vi "HH_Set.vi"(0 "Device List":T3(array[cluster]), 5 "CFD Settings":T2={"Sync Level"=150, "Sync ZeroX"=10, "Sync Offset"=-8000, "Chan Settings"=[{"CHx Level"=50, "CHx ZeroX"=10, "CHx Offset"=350}, {"CHx Level"=50, "CHx ZeroX"=10, "CHx Offset"=50}, {"CHx Level"=150, "CHx ZeroX"=10, "CHx Offset"=19250}, {"CHx Level"=150, "CHx ZeroX"=10, "CHx Offset"=19500}]}, 11 "error in (no error)":errorcluster, 12 "SyncDiv":i32=8, 13 "Offset":i32) -> (3 "ht3 header out":T1={"Comment"="", "Binning"=0, "Offset"=0, "AcquisitionTime (ms)"=0, "HardwareSerial"=0, "SyncDivider"=0, "Resolution (ps)"=0.0, "InpRate0"=0, "InpRate1"=0, "CFD Settings"={"Sync Level"=150, "Sync ZeroX"=10, "Sync Offset"=-1000, "Chan Settings"=[{"CHx Level"=50, "CHx ZeroX"=10, "CHx Offset"=0}, {"CHx Level"=50, "CHx ZeroX"=10, "CHx Offset"=0}, {"CHx Level"=50, "CHx ZeroX"=10, "CHx Offset"=0}, {"CHx Level"=50, "CHx ZeroX"=10, "CHx Offset"=0}]}, "ModuleInfo"=[], "BaseResolution (ps)"=0.0, "RefClockSource"=0, "ChanInfo"=[], "SyncRate"=0, "InputsEnabled"=0}, 6 "Resolution (ps)":dbl, 8 "Range":i32, 10 "Sync Rate":i32, 15 "error out":errorcluster)   [LabVIEW 2010]
uses:
  hhlib.dll
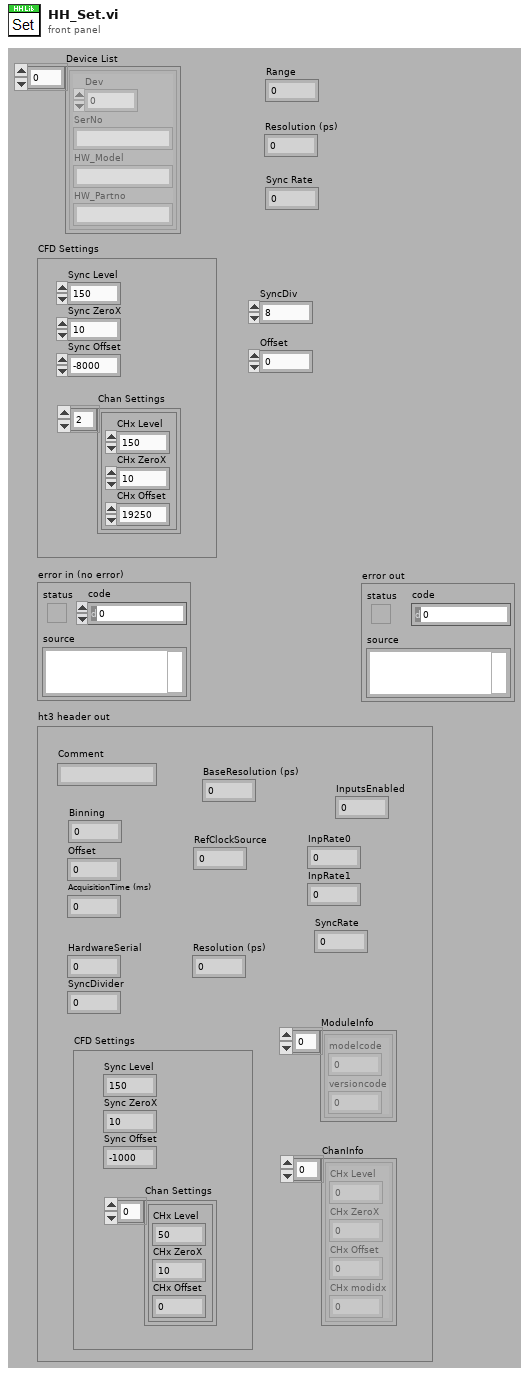
[diagram p1: front panel]
types:
  T1 = cluster{"Comment":string, "Binning":i32, "Offset":i32, "AcquisitionTime (ms)":i32, "HardwareSerial":i32, "SyncDivider":i32, "Resolution (ps)":dbl, "InpRate0":i32, "InpRate1":i32, "CFD Settings":cluster{"Sync Level":i32, "Sync ZeroX":i32, "Sync Offset":i32, "Chan Settings":cluster{"CHx Level":i32, "CHx ZeroX":i32, "CHx Offset":i32}[]}, "ModuleInfo":cluster{"modelcode":i32, "versioncode":i32}[], "BaseResolution (ps)":dbl, "RefClockSource":i32, "ChanInfo":cluster{"CHx Level":i32, "CHx ZeroX":i32, "CHx Offset":i32, "CHx modidx":i32}[], "SyncRate":i32, "InputsEnabled":i64}
  T2 = cluster{"Sync Level":i32, "Sync ZeroX":i32, "Sync Offset":i32, "Chan Settings":cluster{"CHx Level":i32, "CHx ZeroX":i32, "CHx Offset":i32}[]}
  T3 = cluster{"Dev":i32, "SerNo":string, "HW_Model":string, "HW_Partno":string}[]
  T4 = cluster{"CHx Level":i32, "CHx ZeroX":i32, "CHx Offset":i32, "CHx modidx":i32}
  T5 = cluster{"CHx Level":i32, "CHx ZeroX":i32, "CHx Offset":i32}
  T6 = cluster{"CHx Level":i32, "CHx ZeroX":i32, "CHx Offset":i32, "CHx modidx":i32}[]
  T7 = cluster{"CHx Level":i32, "CHx ZeroX":i32, "CHx Offset":i32}[]
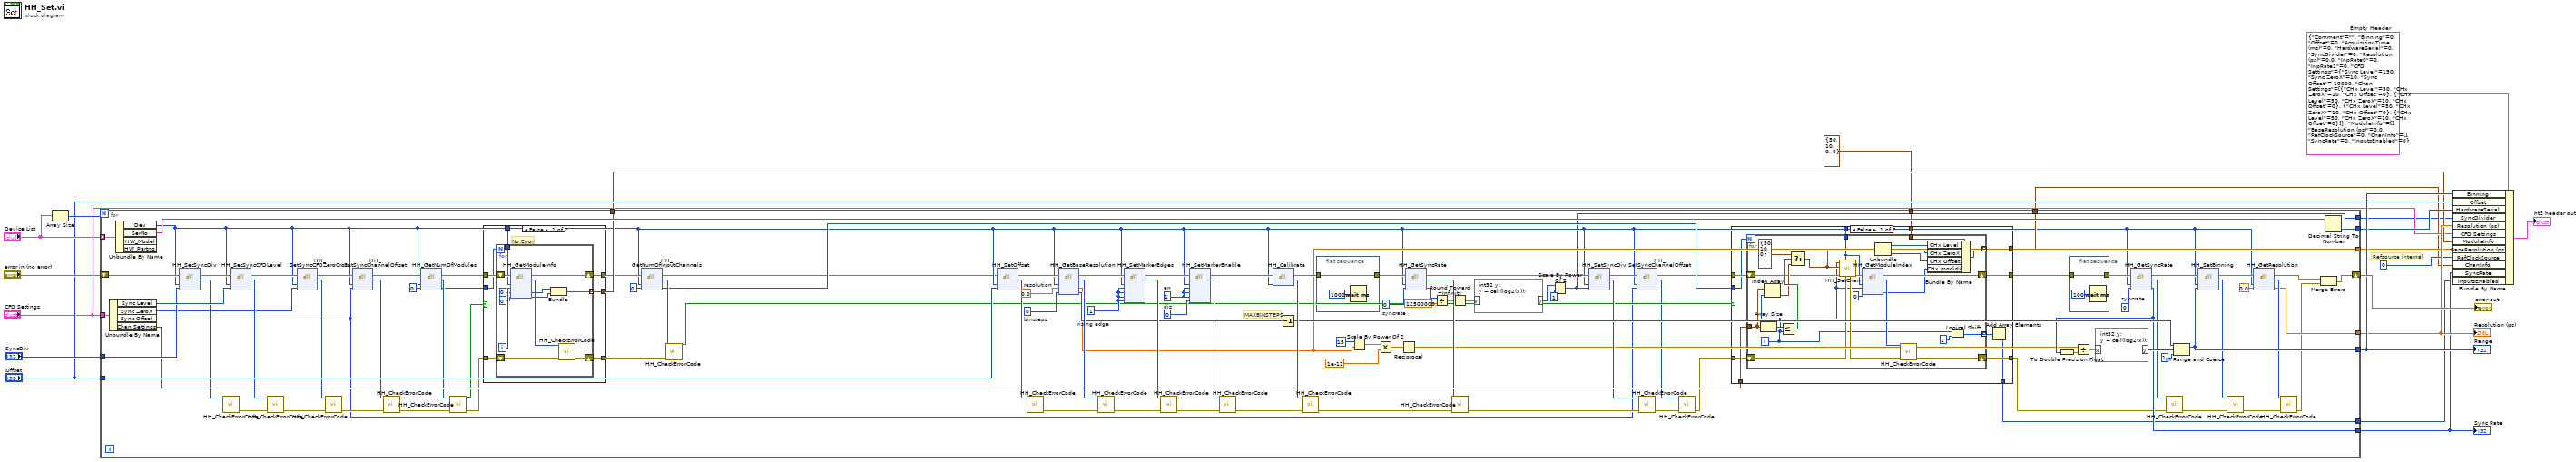
[diagram p0: block diagram]
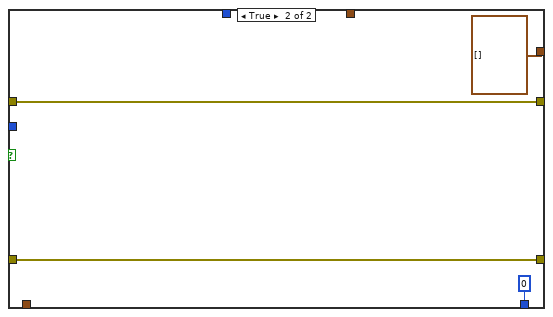
[diagram p2: hidden frame]
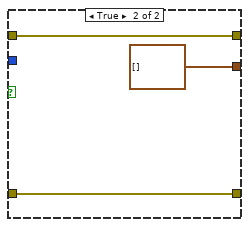
[diagram p3: hidden frame]
diagram:
  w16 = T1 {"Comment"="", "Binning"=0, "Offset"=0, "AcquisitionTime (ms)"=0, "HardwareSerial"=0, "SyncDivider"=0, "Resolution (ps)"=0.0, "InpRate0"=0, "InpRate1"=0, "CFD Settings"={"Sync Level"=150, "Sync ZeroX"=10, "Sync Offset"=-10000, "Chan Settings"=[{"CHx Level"=50, "CHx ZeroX"=10, "CHx Offset"=0}, {"CHx Level"=50, "CHx ZeroX"=10, "CHx Offset"=0}, {"CHx Level"=50, "CHx ZeroX"=10, "CHx Offset"=0}, {"CHx Level"=50, "CHx ZeroX"=10, "CHx Offset"=0}]}, "ModuleInfo"=[], "BaseResolution (ps)"=0.0, "RefClockSource"=0, "ChanInfo"=[], "SyncRate"=0, "InputsEnabled"=0}  # Empty Header
  # "Refsource internal"
  n1 = Array Size(array="Device List") -> (size(s)=w19:i32)
  n2 = for {
    N: w19 -> [_]
    tunnel: "Device List" -> [w129] mode=indexing
    shift-right: [w93] -> w17
    shift-left: "error in (no error)" -> [w118]
    tunnel: "CFD Settings" -> [w122]
    tunnel: "SyncDiv" -> [w120]
    tunnel: "Offset" -> [w119]
    tunnel: [w111] -> w14
    tunnel: [w80] -> w10
    tunnel: [w72] -> w3
    tunnel: [w90] -> w11
    tunnel: [w52] -> w9
    tunnel: [w51] -> w8
    tunnel: [w37] -> w4
    tunnel: T4 {"CHx Level"=50, "CHx ZeroX"=10, "CHx Offset"=0, "CHx modidx"=0} ("element") -> [w36]
    tunnel: [w35] -> w2
    tunnel: [w21] -> w1
    w47 = 0  # dis
    w48 = 1  # en
    w73 = 0  # syncrate
    w85 = 0  # syncrate
    w86 = 0  # binsteps
    w87 = 0.0  # resolution
    w123 = 1  # rising edge
    # "MAXBINSTEPS"
    n3 = Unbundle By Name(w122) -> ("Sync Level"=w121:i32, "Sync ZeroX"=w89:i32, "Sync Offset"=w30:i32, "Chan Settings"=w88:T7)
    n4 = Unbundle By Name(w129) -> ("Dev"=w31:i32, "SerNo"=w91:string)  [unwired: 2 out]
    n5 = dll-call lib="C:/LabVIEW Programs/MT Scan/SubVIs/hhlib.dll" fn="HH_SetSyncDiv"(error in=w118, "devidx"=w31, "div"=w120) -> (error out=w128:errorcluster, "return type"=w109:i32)  [unwired: 4 in, 1 out]
    n6 = call "HH_CheckErrorCode.vi"("errcode"=w109) -> ("error out"=w108:errorcluster)  [unwired: 13 in, 1 out]
    n7 = dll-call lib="C:/LabVIEW Programs/MT Scan/SubVIs/hhlib.dll" fn="HH_SetSyncCFDLevel"(error in=w128, "devidx"=w31, "value"=w121) -> (error out=w127:errorcluster, "return type"=w107:i32)  [unwired: 4 in, 1 out]
    n8 = call "HH_CheckErrorCode.vi"("errcode"=w107, "error in (no error)"=w108) -> ("error out"=w106:errorcluster)  [unwired: 12 in, 1 out]
    n9 = dll-call lib="C:/LabVIEW Programs/MT Scan/SubVIs/hhlib.dll" fn="HH_SetSyncCFDZeroCross" label="HH_SetSyncZeroX"(error in=w127, "devidx"=w31, "value"=w89) -> (error out=w126:errorcluster, "return type"=w105:i32)  [unwired: 4 in, 1 out]
    n10 = call "HH_CheckErrorCode.vi"("errcode"=w105, "error in (no error)"=w106) -> ("error out"=w103:errorcluster)  [unwired: 12 in, 1 out]
    n11 = dll-call lib="C:/LabVIEW Programs/MT Scan/SubVIs/hhlib.dll" fn="HH_SetSyncChannelOffset" label="HH_SetSyncChOffset"(error in=w126, "devidx"=w31, "value"=w30) -> (error out=w54:errorcluster, "return type"=w104:i32)  [unwired: 4 in, 1 out]
    n12 = call "HH_CheckErrorCode.vi"("errcode"=w104, "error in (no error)"=w103) -> ("error out"=w55:errorcluster)  [unwired: 12 in, 1 out]
    n13 = dll-call lib="C:/LabVIEW Programs/MT Scan/SubVIs/hhlib.dll" fn="HH_GetNumOfModules"(error in=w54, "devidx"=w31, "nummod"=0) -> (error out=w57:errorcluster, "return type"=w59:i32, "nummod"=w56:i32)  [unwired: 3 in, 1 out]
    n14 = call "HH_CheckErrorCode.vi"("errcode"=w59, "error in (no error)"=w55) -> ("Is Error"=w58:bool, "error out"=w53:errorcluster)  [unwired: 12 in]
    n15 = case shown="False" w58 {
      tunnel: w57 -> [w175 w190]
      tunnel: [w174 w190] -> w43
      tunnel: w56 -> [w173 _]
      tunnel: w53 -> [w172 w189]
      tunnel: [w171 w189] -> w42
      tunnel: w31 -> [w170 _]
      tunnel: [w169 cluster{"modelcode":i32, "versioncode":i32}[] []] -> w52
      frame False {
        # "No Error"
        n16 = for {
          N: w173 -> [_]
          shift-right: [w179] -> w174
          shift-left: w175 -> [w187]
          shift-right: [w185] -> w171
          shift-left: w172 -> [w186]
          tunnel: w170 -> [w183]
          tunnel: [w176] -> w169 mode=indexing
          i -> [w182]
          n17 = dll-call lib="C:/LabVIEW Programs/MT Scan/SubVIs/hhlib.dll" fn="HH_GetModuleInfo"(error in=w187, "devidx"=w183, "modidx"=w182, "modelcode"=0, "versioncode"=0) -> (error out=w179:errorcluster, "return type"=w184:i32, "modelcode"=w178:i32, "versioncode"=w177:i32)  [unwired: 4 in, 1 out]
          n18 = Bundle("modelcode"=w178, "versioncode"=w177) -> (w176:cluster{"modelcode":i32, "versioncode":i32})  [unwired: 1 in]
          n19 = call "HH_CheckErrorCode.vi"("errcode"=w184, "error in (no error)"=w186) -> ("error out"=w185:errorcluster)  [unwired: 12 in, 1 out]
        }
      }
      frame True {
      }
    }
    n20 = dll-call lib="C:/LabVIEW Programs/MT Scan/SubVIs/hhlib.dll" fn="HH_GetNumOfInputChannels"(error in=w43, "devidx"=w31, "nchannels"=0) -> (error out=w25:errorcluster, "return type"=w41:i32, "nchannels"=w38:i32)  [unwired: 3 in, 1 out]
    n21 = call "HH_CheckErrorCode.vi"("errcode"=w41, "error in (no error)"=w42) -> ("Is Error"=w40:bool)  [unwired: 12 in, 1 out]
    n22 = dll-call lib="C:/LabVIEW Programs/MT Scan/SubVIs/hhlib.dll" fn="HH_SetOffset"(error in=w25, "devidx"=w31, "offset"=w119) -> (error out=w125:errorcluster, "return type"=w102:i32)  [unwired: 4 in, 1 out]
    n23 = call "HH_CheckErrorCode.vi"("errcode"=w102) -> ("error out"=w101:errorcluster)  [unwired: 13 in, 1 out]
    n24 = dll-call lib="C:/LabVIEW Programs/MT Scan/SubVIs/hhlib.dll" fn="HH_GetBaseResolution"(error in=w125, "devidx"=w31, "resolution"=w87, "binsteps"=w86) -> (error out=w124:errorcluster, "return type"=w92:i32, "resolution"=w51:dbl, "binsteps"=w83:i32)  [unwired: 3 in, 1 out]
    n25 = call "HH_CheckErrorCode.vi"("errcode"=w92, "error in (no error)"=w101) -> ("error out"=w100:errorcluster)  [unwired: 12 in, 1 out]
    n26 = dll-call lib="C:/LabVIEW Programs/MT Scan/SubVIs/hhlib.dll" fn="HH_SetMarkerEdges"(error in=w124, "devidx"=w31, "me0"=w123, "me1"=w123, "me2"=w123, "me3"=w123) -> (error out=w50:errorcluster, "return type"=w99:i32)  [unwired: 7 in, 1 out]
    n27 = call "HH_CheckErrorCode.vi"("errcode"=w99, "error in (no error)"=w100) -> ("error out"=w46:errorcluster)  [unwired: 12 in, 1 out]
    n28 = dll-call lib="C:/LabVIEW Programs/MT Scan/SubVIs/hhlib.dll" fn="HH_SetMarkerEnable"(error in=w50, "devidx"=w31, "en0"=w48, "en1"=w48, "en2"=w48, "en3"=w47) -> (error out=w49:errorcluster, "return type"=w44:i32)  [unwired: 7 in, 1 out]
    n29 = call "HH_CheckErrorCode.vi"("errcode"=w44, "error in (no error)"=w46) -> ("error out"=w45:errorcluster)  [unwired: 12 in, 1 out]
    n30 = dll-call lib="C:/LabVIEW Programs/MT Scan/SubVIs/hhlib.dll" fn="HH_Calibrate"(error in=w49, "devidx"=w31) -> (error out=w117:errorcluster, "return type"=w98:i32)  [unwired: 3 in, 1 out]
    n31 = Decrement(x=w83) -> (x-1=w82:i32)
    n32 = call "HH_CheckErrorCode.vi"("errcode"=w98, "error in (no error)"=w45) -> ("error out"=w97:errorcluster)  [unwired: 12 in, 1 out]
    n33 = flat-sequence {
      tunnel: w117 -> [w194]
      tunnel: [w194] -> w116
      frame #0 {
        n34 = Wait (ms)(milliseconds to wait=u32 1000) -> ()  [unwired: 1 out]
      }
    }
    n35 = Scale By Power Of 2(n=15, x=w51) -> (x*2^n=w66:dbl)
    n36 = Multiply(x=w66, y=1e-12) -> (x*y=w64:dbl)
    n37 = Reciprocal(x=w64) -> (1/x=w63:dbl)
    n38 = dll-call lib="C:/LabVIEW Programs/MT Scan/SubVIs/hhlib.dll" fn="HH_GetSyncRate"(error in=w116, "devidx"=w31, "syncrate"=w85) -> (error out=w79:errorcluster, "return type"=w84:i32, "syncrate"=w78:i32)  [unwired: 3 in, 1 out]
    n39 = Divide(x=w78, y=12500000.0) -> (x/y=w76:dbl)
    n40 = call "HH_CheckErrorCode.vi"("errcode"=w84, "error in (no error)"=w97) -> ("error out"=w69:errorcluster)  [unwired: 12 in, 1 out]
    n41 = Round Toward +Infinity(x=w76) -> (ceil(x): smallest int >= x=w24:dbl)
    n42 = formula code="int32 y;\ny = ceil(log2(x));"("x"=w24) -> ("y"=w23:i32)
    n43 = Scale By Power Of 2(n=w23, x=1) -> (x*2^n=w21:i32)
    n44 = dll-call lib="C:/LabVIEW Programs/MT Scan/SubVIs/hhlib.dll" fn="HH_SetSyncDiv"(error in=w79, "devidx"=w31, "div"=w21) -> (error out=w34:errorcluster, "return type"=w71:i32)  [unwired: 4 in, 1 out]
    n45 = dll-call lib="C:/LabVIEW Programs/MT Scan/SubVIs/hhlib.dll" fn="HH_SetSyncChannelOffset" label="HH_SetSyncChOffset"(error in=w34, "devidx"=w31, "value"=w30) -> (error out=w26:errorcluster, "return type"=w32:i32)  [unwired: 4 in, 1 out]
    n46 = call "HH_CheckErrorCode.vi"("errcode"=w71, "error in (no error)"=w69) -> ("error out"=w33:errorcluster)  [unwired: 12 in, 1 out]
    n47 = call "HH_CheckErrorCode.vi"("errcode"=w32, "error in (no error)"=w33) -> ("error out"=w29:errorcluster)  [unwired: 12 in, 1 out]
    n48 = case shown="False" w40 {
      tunnel: w88 -> [w140 _]
      tunnel: [w139 w168] -> w27
      tunnel: [w138 w167] -> w28
      tunnel: w26 -> [w137 w168]
      tunnel: w31 -> [w136 _]
      tunnel: w29 -> [w135 w167]
      tunnel: w38 -> [w134 _]
      tunnel: [w133 T6 []] -> w37
      tunnel: w36 -> [w132 _]
      tunnel: [w130 i64 0] -> w35
      frame False {
        n49 = for {
          N: w134 -> [_]
          tunnel: w140 -> [w163]
          tunnel: w136 -> [w155]
          shift-right: [w156] -> w139
          shift-left: w137 -> [w159]
          shift-right: [w152] -> w138
          shift-left: w135 -> [w158]
          tunnel: [w149] -> w133 mode=indexing
          tunnel: w132 -> [w150]
          tunnel: [w141] -> w131 mode=indexing
          i -> [w143]
          n50 = Array Size(array=w163) -> (size(s)=w164:i32)
          n51 = Index Array(array=w163, index=w143) -> (element=w160:T5)
          n52 = Less Or Equal?(x=w164, y=w143) -> (x <= y?=w162:bool)
          n53 = Select(t=T5 {"CHx Level"=50, "CHx ZeroX"=10, "CHx Offset"=0} ("element"), s=w162, f=w160) -> (s? t:f=w147:T5)
          n54 = call "HH_SetChan.vi"("error in 2"=w158, "Dev"=w155, "error in"=w159, "CHx CFD Settings"=w147, "Chan"=w143) -> ("error out"=w157:errorcluster, "error out 2"=w153:errorcluster)  [unwired: 5 in]
          n55 = dll-call lib="C:/LabVIEW Programs/MT Scan/SubVIs/hhlib.dll" fn="HH_GetModuleIndex"(error in=w157, "devidx"=w155, "channel"=w143, "modidx"=0) -> (error out=w156:errorcluster, "return type"=w151:i32, "modidx"=w148:i32)  [unwired: 4 in, 1 out]
          n56 = Unbundle(w147) -> ("CHx Level"=w146:i32, "CHx ZeroX"=w144:i32, "CHx Offset"=w145:i32)
          n57 = call "HH_CheckErrorCode.vi"("errcode"=w151, "error in (no error)"=w153) -> ("error out"=w152:errorcluster)  [unwired: 12 in, 1 out]
          n58 = Bundle By Name(cluster=w150, "CHx Level"=w146, "CHx ZeroX"=w144, "CHx Offset"=w145, "CHx modidx"=w148) -> (w149:T4)
          n59 = Logical Shift(y=w143, x=i64 1) -> (x << y=w141:i64)
        }
        n60 = Add Array Elements(numeric array=w131) -> (sum=w130:i64)
      }
      frame True {
      }
    }
    n61 = flat-sequence {
      tunnel: w27 -> [w192]
      tunnel: [w192] -> w75
      frame #0 {
        n62 = Wait (ms)(milliseconds to wait=u32 100) -> ()  [unwired: 1 out]
      }
    }
    n63 = dll-call lib="C:/LabVIEW Programs/MT Scan/SubVIs/hhlib.dll" fn="HH_GetSyncRate"(error in=w75, "devidx"=w31, "syncrate"=w73) -> (error out=w74:errorcluster, "return type"=w70:i32, "syncrate"=w72:i32)  [unwired: 3 in, 1 out]
    n64 = To Double Precision Float(number=w72) -> (double precision float=w113:dbl)
    n65 = Divide(x=w63, y=w113) -> (x/y=w115:dbl)
    n66 = formula code="int32 y;\ny = ceil(log2(x));"("x"=w115) -> ("y"=w112:i32)
    n67 = call "HH_CheckErrorCode.vi"("errcode"=w70, "error in (no error)"=w28) -> ("error out"=w68:errorcluster)  [unwired: 12 in, 1 out]
    n68 = In Range and Coerce(upper limit=w82, x=w112, lower limit=1) -> (coerced(x)=w111:i32)  [unwired: 1 out]
    n69 = dll-call lib="C:/LabVIEW Programs/MT Scan/SubVIs/hhlib.dll" fn="HH_SetBinning"(error in=w74, "devidx"=w31, "binning"=w111) -> (error out=w114:errorcluster, "return type"=w96:i32)  [unwired: 4 in, 1 out]
    n70 = call "HH_CheckErrorCode.vi"("errcode"=w96, "error in (no error)"=w68) -> ("error out"=w95:errorcluster)  [unwired: 12 in, 1 out]
    n71 = dll-call lib="C:/LabVIEW Programs/MT Scan/SubVIs/hhlib.dll" fn="HH_GetResolution"(error in=w114, "devidx"=w31, "resolution"=0.0) -> (error out=w62:errorcluster, "return type"=w94:i32, "resolution"=w80:dbl)  [unwired: 3 in, 1 out]
    n72 = call "HH_CheckErrorCode.vi"("errcode"=w94, "error in (no error)"=w95) -> ("error out"=w61:errorcluster)  [unwired: 12 in, 1 out]
    n73 = Merge Errors(w62, w61) -> (w93:errorcluster)
    n74 = Decimal String To Number(string=w91) -> (number=w90:i32)  [unwired: 2 in, 1 out]
  }
  "error out" <- w17
  "Range" <- w14
  "Resolution (ps)" <- w10
  "Sync Rate" <- w3
  n75 = Bundle By Name(cluster=w16, "Binning"=w14, "Offset"="Offset", "HardwareSerial"=w11, "SyncDivider"=w1, "Resolution (ps)"=w10, "CFD Settings"="CFD Settings", "ModuleInfo"=w9, "BaseResolution (ps)"=w8, "RefClockSource"=0 ("refsource"), "ChanInfo"=w4, "SyncRate"=w3, "InputsEnabled"=w2) -> (→"ht3 header out":T1)
